vi "Uninitialise.vi"(8 "Error In":errorcluster) -> (0 "Error Out":errorcluster)   [LabVIEW 2012]
uses:
  <vilib>/robotics/Simulator/NI_Robotics_Simulator.lvlib
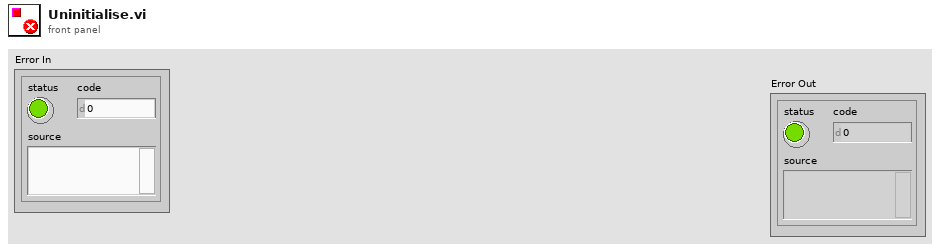
[diagram p1: front panel]
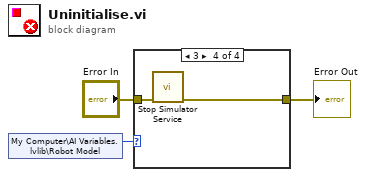
[diagram p0: block diagram]
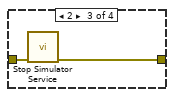
[diagram p4: hidden frame]
diagram:
  n1 = shared-variable "My Computer\\AI Variables.lvlib\\Robot Model"() -> (w3:u16)  [unwired: 1 in, 1 out]
  n2 = case shown="3" w3 {
    tunnel: [w4 w5 w6 w8] -> w2
    tunnel: "Error In" -> [w4 w5 w7 w9]
    frame 0, Default {
    }
    frame 1 {
    }
    frame 2 {
      n3 = call <vilib>:"Stop Simulator Service.vi"("error in (no error)"=w7) -> ("error out"=w6:errorcluster)  [unwired: 10 in]
    }
    frame 3 {
      n4 = call <vilib>:"Stop Simulator Service.vi"("error in (no error)"=w9) -> ("error out"=w8:errorcluster)  [unwired: 10 in]
    }
  }
  "Error Out" <- w2
